vi "setValvesPuffedArduinoNew.vi"(7 "valve data puffed":bool[](array[boolean])=[FALSE, FALSE, FALSE, FALSE, FALSE, FALSE, FALSE, FALSE], 8 "valve data close":bool[](array[boolean])=[FALSE, FALSE, FALSE, FALSE, FALSE, FALSE, FALSE, FALSE], 9 "valve data open":bool[](array[boolean])=[FALSE, FALSE, FALSE, FALSE, FALSE, FALSE, FALSE, FALSE], 10 "milliseconds to wait":u32=1000, 11 "numPuffs":i32=2) -> ()   [LabVIEW 2012]
uses:
  GlobalValves.vi
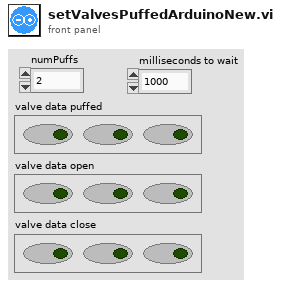
[diagram p1: front panel]
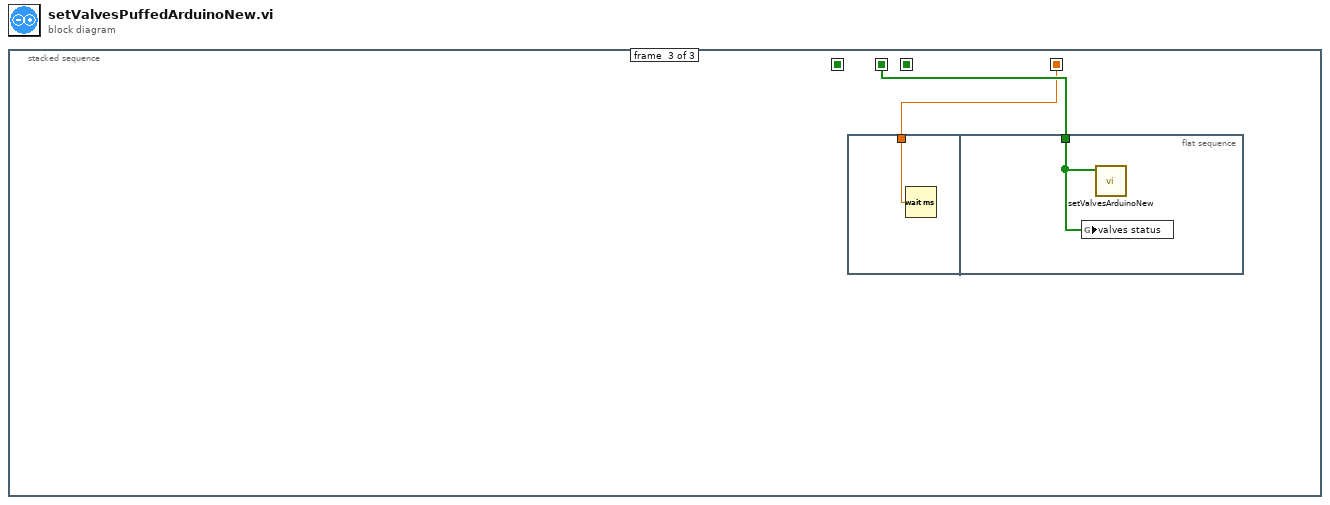
[diagram p0: block diagram]
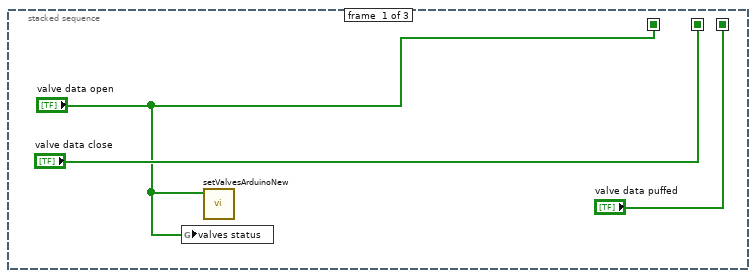
[diagram p2: hidden frame]
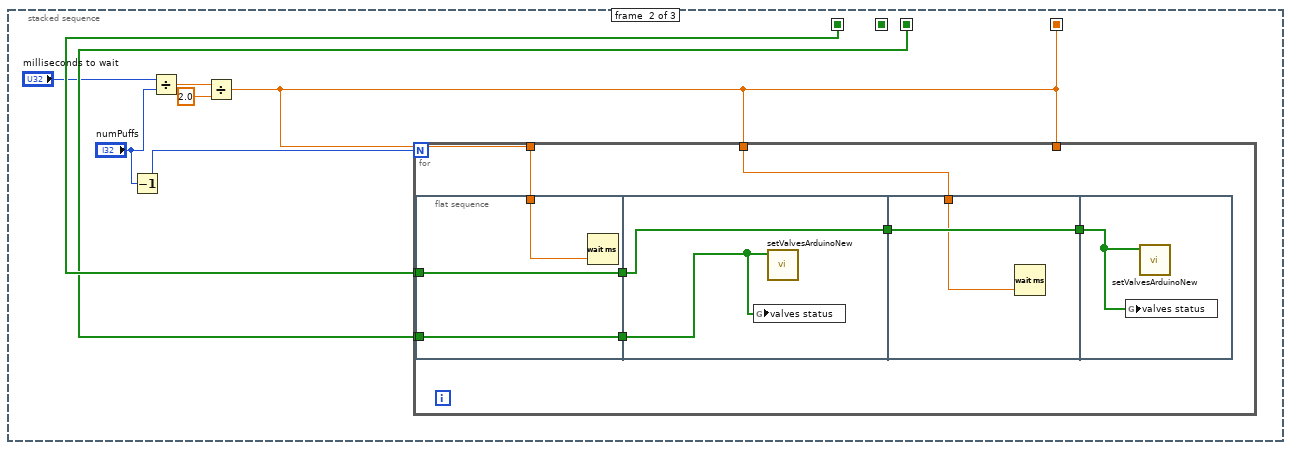
[diagram p3: hidden frame]
diagram:
  n1 = stacked-sequence {
    seq-local: ["valve data open" _ _] -> [_ w9 _]
    seq-local: ["valve data close" _ _] -> [_ _ w29]
    seq-local: ["valve data puffed" _ _] -> [_ w8 _]
    seq-local: [_ w7 _] -> [_ _ w28]
    frame #0 {
      n2 = global write "GlobalValves.vi" "valves status"("valve data open") -> ()
      n3 = call "setValvesArduinoNew.vi"("valve data"="valve data open") -> ()  [unwired: 11 in]
    }
    frame #1 {
      n4 = Decrement(x="numPuffs") -> (x-1=w4:i32)
      n5 = Divide(x="milliseconds to wait", y="numPuffs") -> (x/y=w10:dbl)
      n6 = Divide(x=w10, y=2.0) -> (x/y=w7:dbl)
      n7 = for {
        N: w4 -> [_]
        tunnel: w9 -> [w19]
        tunnel: w8 -> [w18]
        tunnel: w7 -> [w15]
        tunnel: w7 -> [_]
        tunnel: w7 -> [w12]
        n8 = flat-sequence {
          tunnel: w18 -> [w21]
          tunnel: w19 -> [w22]
          tunnel: [w22] -> w14
          tunnel: [w21] -> w13
          tunnel: w12 -> [w20]
          tunnel: [w23] -> w16
          tunnel: w14 -> [w23]
          tunnel: w13 -> [w24]
          tunnel: [w26] -> w17
          tunnel: w16 -> [w26]
          tunnel: w15 -> [w25]
          tunnel: w17 -> [w27]
          frame #0 {
            n9 = Wait (ms)(milliseconds to wait=w20) -> ()  [unwired: 1 out]
          }
          frame #1 {
            n10 = global write "GlobalValves.vi" "valves status"(w24) -> ()
            n11 = call "setValvesArduinoNew.vi"("valve data"=w24) -> ()  [unwired: 11 in]
          }
          frame #2 {
            n12 = Wait (ms)(milliseconds to wait=w25) -> ()  [unwired: 1 out]
          }
          frame #3 {
            n13 = global write "GlobalValves.vi" "valves status"(w27) -> ()
            n14 = call "setValvesArduinoNew.vi"("valve data"=w27) -> ()  [unwired: 11 in]
          }
        }
      }
    }
    frame #2 {
      n15 = flat-sequence {
        tunnel: w28 -> [w30]
        tunnel: w29 -> [w31]
        frame #0 {
          n16 = Wait (ms)(milliseconds to wait=w30) -> ()  [unwired: 1 out]
        }
        frame #1 {
          n17 = global write "GlobalValves.vi" "valves status"(w31) -> ()
          n18 = call "setValvesArduinoNew.vi"("valve data"=w31) -> ()  [unwired: 11 in]
        }
      }
    }
  }
